vi "MeasureAtFreq.vi"(8 "error in (no error)":errorcluster, 10 "Frequency (Hz)":dbl, 11 "SpecA_MXA in":refnum<class "SpecA_MXA.lvclass">) -> (0 "error out":errorcluster, 2 "Power (dBm)":dbl, 3 "SpecA_MXA out":refnum<class "SpecA_MXA.lvclass">)   [LabVIEW 2014, in "SpecA_MXA.lvclass"]
uses:
  SpecA_MXA.lvclass
  SpecA_MXA.lvclass/SpecA_MXA.ctl
  data/Agilent MXA Series/Configure Frequency (Center Span).vi
  data/Read Trace (Swept SA).vi
  data/NI_AALBase.lvlib
  data/Agilent MXA Series.lvlib
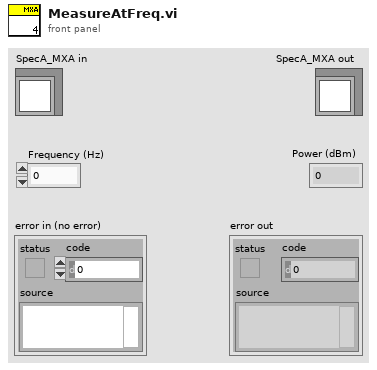
[diagram p1: front panel]
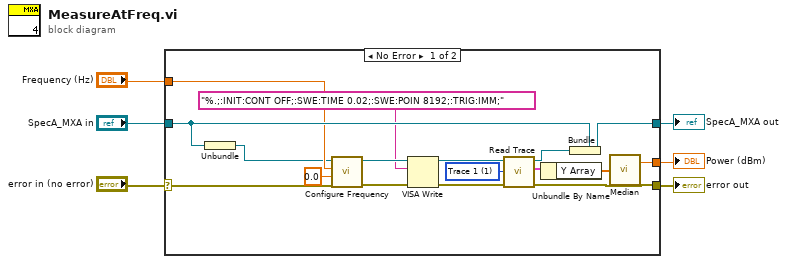
[diagram p0: block diagram]
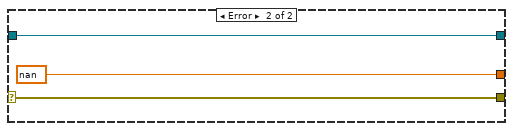
[diagram p2: hidden frame]
diagram:
  n1 = case shown="No Error" "error in (no error)" {
    selector: "error in (no error)" -> [w7 w25]
    tunnel: "Frequency (Hz)" -> [w20 _]
    tunnel: "SpecA_MXA in" -> [w21 w26]
    tunnel: [w15 w25] -> w3
    tunnel: [w23 nan ("Amplitude (Cal)")] -> w2
    tunnel: [w22 w26] -> w1
    frame No Error {
      w14 = 1 items=["Trace 1"=1, "Trace 2"=2, "Trace 3"=3, "Trace 4"=4] ("Trace Name (1: Trace 1)")
      n2 = Unbundle(w21) -> (w8:refnum<visa-resource-name>)
      n3 = call-poly "Configure Frequency.vi"("error in (no error)"=w7, "Span (2.65E+10 Hz)"=0.0, "Center Frequency (1.325E+10 Hz)"=w20, "VISA resource name"=w8) -> ("error out"=w12:errorcluster, "VISA resource name out"=w13:refnum<visa-resource-name>)  [unwired: 6 in]
      n4 = VISA Write(VISA resource name=w13, write buffer="%.;:INIT:CONT OFF;:SWE:TIME 0.02;:SWE:POIN 8192;:TRIG:IMM;" ("format string"), error in (no error)=w12) -> (VISA resource name out=w10:refnum<visa-resource-name>, error out=w11:errorcluster)  [unwired: 1 out]
      n5 = call-poly "Read Trace.vi"("error in (no error)"=w11, "Trace Name (1: Trace 1)"=w14, "VISA resource name"=w10) -> ("error out"=w15:errorcluster, "Trace Waveform"=w18:cluster{"X Array":dbl[], "Y Array":dbl[]}, "VISA resource name out"=w17:refnum<visa-resource-name>)  [unwired: 6 in]
      n6 = Unbundle By Name(w18) -> ("Y Array"=w16:dbl[])
      n7 = Bundle(cluster=w21, w17) -> (w22:refnum<class "SpecA_MXA.lvclass">)
      n8 = call "Median.vi"("X"=w16) -> ("median"=w23:dbl)  [unwired: 1 out]
    }
    frame Error {
    }
  }
  "error out" <- w3
  "SpecA_MXA out" <- w1
  "Power (dBm)" <- w2
